vi "Drop Oneof Constant into Case Structure Default.vi"(8 "error in (no error)":errorcluster, 9 "Oneof Container Name":string, 10 "CaseStructure in":refnum<vi>, 11 "Library in":refnum<vi>) -> (0 "error out":errorcluster, 1 "LVClass Constant Terminal out":refnum<vi>, 2 "CaseStructure out":refnum<vi>, 3 "Library item out":refnum<vi>)   [LabVIEW 2019, in "gRPC Template Creation Utility.lvlib"]
uses:
  gRPC Template Creation Utility.lvlib
  <vilib>/Utility/miscctls.llb/LVPointTypeDef.ctl
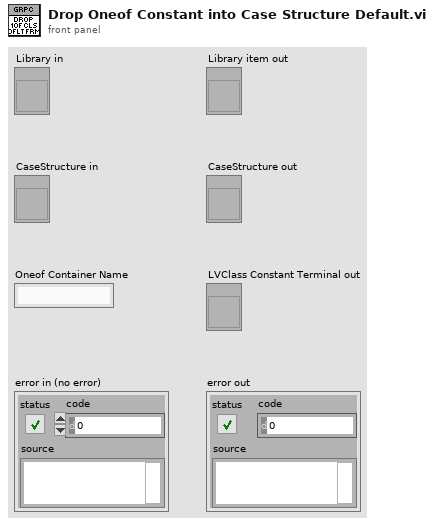
[diagram p1: front panel]
types:
  T1 = typedef "LVPointTypeDef.ctl" = cluster{"Horizontal":i16, "Vertical":i16}
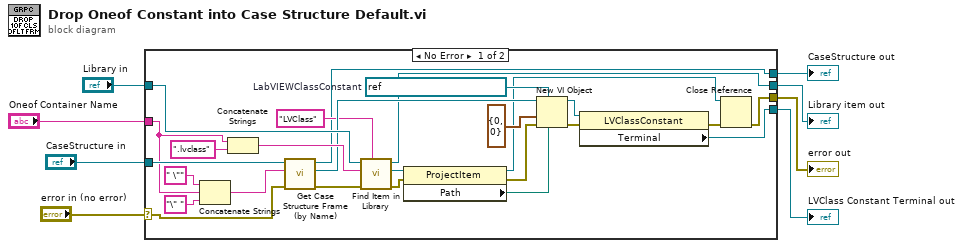
[diagram p0: block diagram]
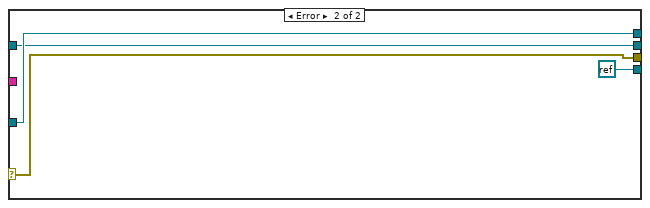
[diagram p2: hidden frame]
diagram:
  n1 = case shown="No Error" "error in (no error)" {
    selector: "error in (no error)" -> [w12 w37]
    tunnel: "CaseStructure in" -> [w34 w38]
    tunnel: "Oneof Container Name" -> [w30 _]
    tunnel: "Library in" -> [w28 w36]
    tunnel: [w21 refnum<k0> refnum] -> w5
    tunnel: [w15 w37] -> w4
    tunnel: [w14 w36] -> w3
    tunnel: [w13 w38] -> w2
    frame No Error {
      w33 = refnum<vi> refnum  # LabVIEWClassConstant
      n2 = Concatenate Strings(" \"" ("string"), w30, "\" " ("string")) -> (w11:string)
      n3 = Concatenate Strings(w30, ".lvclass" ("Item Name")) -> (w31:string)
      n4 = call "Get Case Structure Frame (by Name).vi"("error in (no error)"=w12, "element"=w11, "CaseStructure in"=w34) -> ("error out"=w19:errorcluster, "Frame ref out"=w26:refnum<vi>, "CaseStructure out"=w13:refnum<vi>)  [unwired: 5 in, 1 out]
      n5 = call "Find Item in Library.vi"("Item Type"="LVClass", "error in (no error)"=w19, "Item Name"=w31, "Library item in"=w28) -> ("error out"=w20:errorcluster, "Project Item (Library Item)"=w29:refnum<vi>, "Library item out"=w14:refnum<vi>)  [unwired: 4 in, 1 out]
      n6 = property class="ProjectItem"(reference=w29, error in=w20) -> (reference out=w17:refnum<vi>, error out=w18:errorcluster, "Path"=w27:path)
      n7 = New VI Object(vi object class=w33, owner refnum=w26, position/next to=T1 {"Horizontal"=0, "Vertical"=0} ("location"), 6:w27, 8:w18) -> (object refnum=w23:refnum<vi>, 0:w22:errorcluster)  [unwired: 3 in]
      n8 = property class="LVClassConstant"(reference=w23, error in=w22) -> (error out=w16:errorcluster, "Terminal"=w21:refnum<vi>)  [unwired: 1 out]
      n9 = Close Reference(reference=w17, error in (no error)=w16) -> (error out=w15:errorcluster)
    }
    frame Error {
    }
  }
  "LVClass Constant Terminal out" <- w5
  "error out" <- w4
  "Library item out" <- w3
  "CaseStructure out" <- w2
